vi "Main - Handle Flat BOM Drag&Drop.vi"(8 "error in (no error)":errorcluster, 10 "Drag&Drop Data":T2, 11 "TreeControl in":refnum<vi>) -> (0 "error out":errorcluster, 2 "Data":T1, 3 "Refresh Table":bool)   [LabVIEW 2018]
uses:
  TypeDef/Main - Handle Heirarchy Drag&Drop - Data.ctl
  TypeDef/Main - Handle Heirarchy Drag&Drop - States.ctl
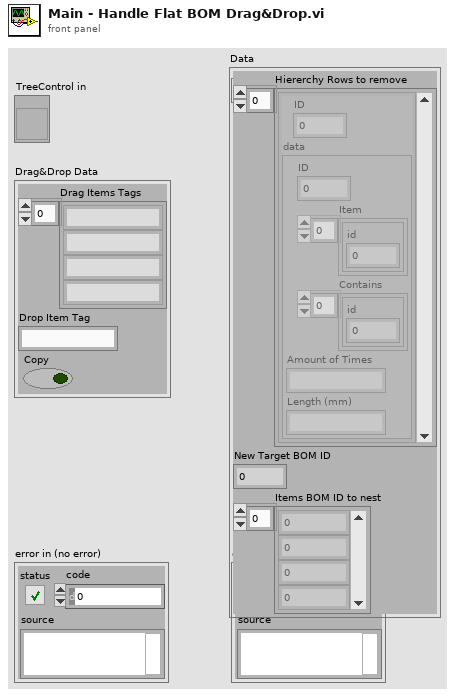
[diagram p1: front panel]
types:
  T1 = typedef "Main - Handle Heirarchy Drag&Drop - Data.ctl" = cluster{"Hiererchy Rows to remove":cluster{"ID":i32, "data":cluster{"ID":i32, "Item":cluster{"id":i32}[], "Contains":cluster{"id":i32}[], "Amount of Times":string, "Length (mm)":string}}[], "New Target BOM ID":i32, "Items BOM ID to nest":i32[]}
  T2 = cluster{"Drag Items Tags":string[], "Drop Item Tag":string, "Copy":bool}
  T3 = typedef "Main - Handle Heirarchy Drag&Drop - States.ctl" = enum16{"Check Data", "GET previous container entries", "Remove container entries", "Create new container entries", "Restore container entries", "Report Error", "Exit"}
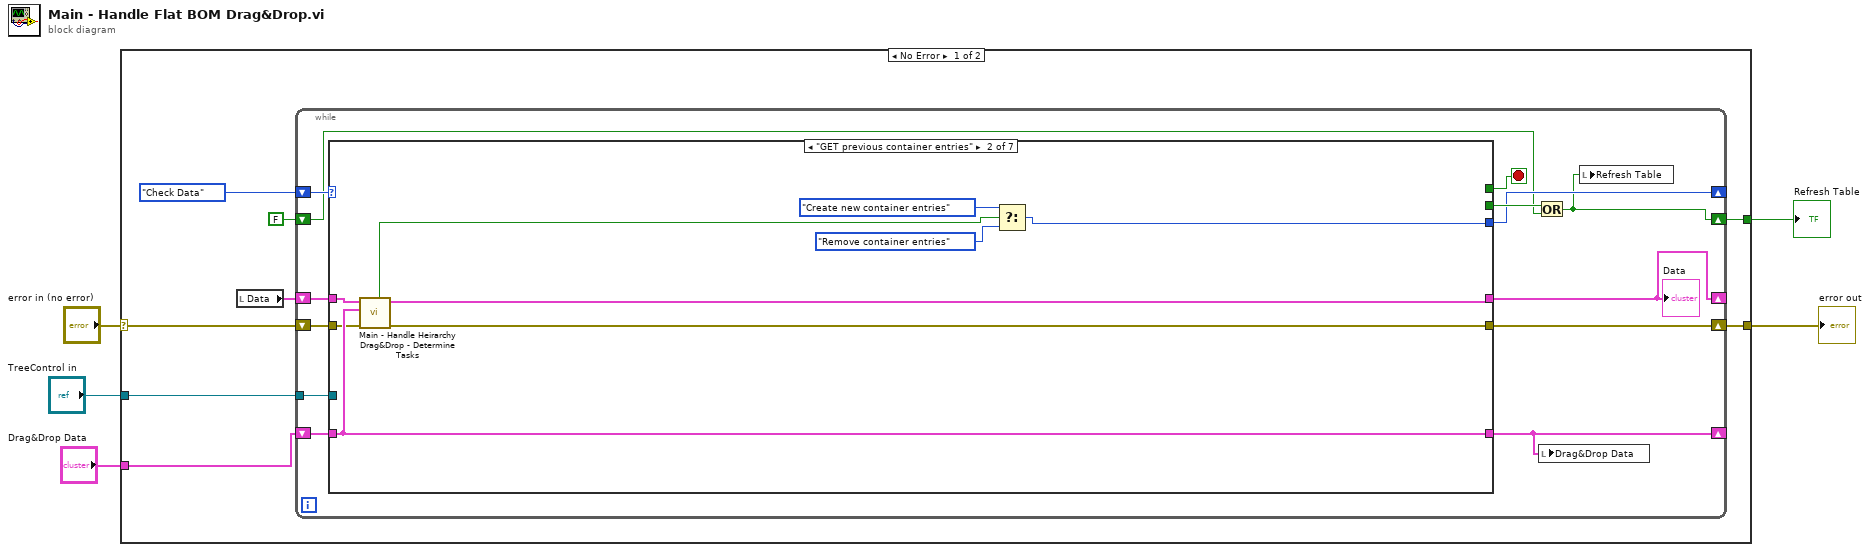
[diagram p0: block diagram]
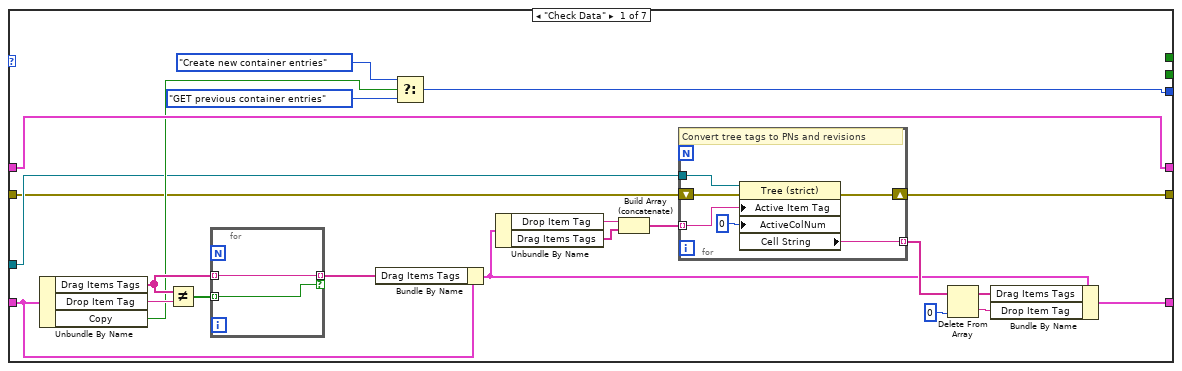
[diagram p2: hidden frame]
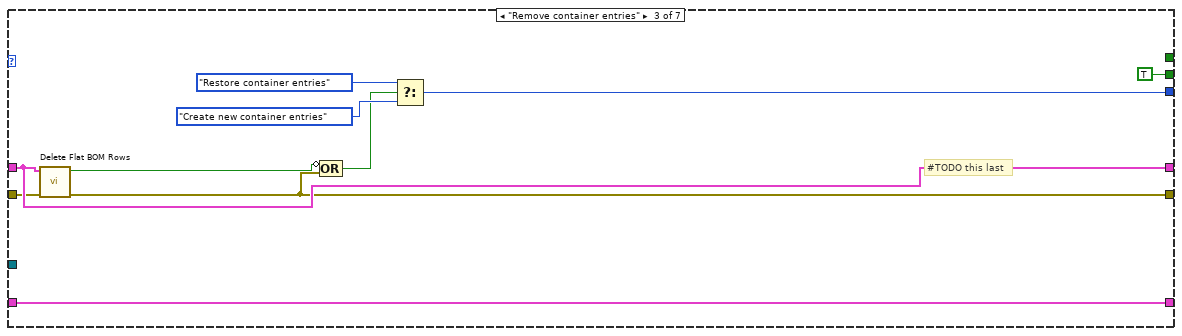
[diagram p3: hidden frame]
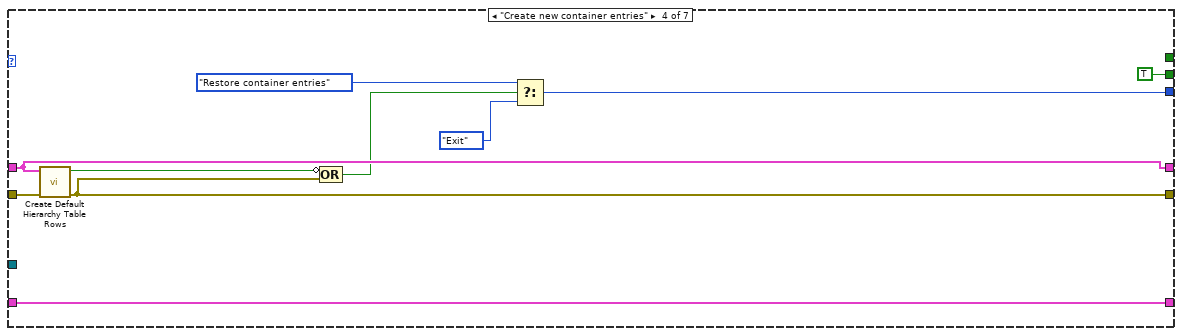
[diagram p4: hidden frame]
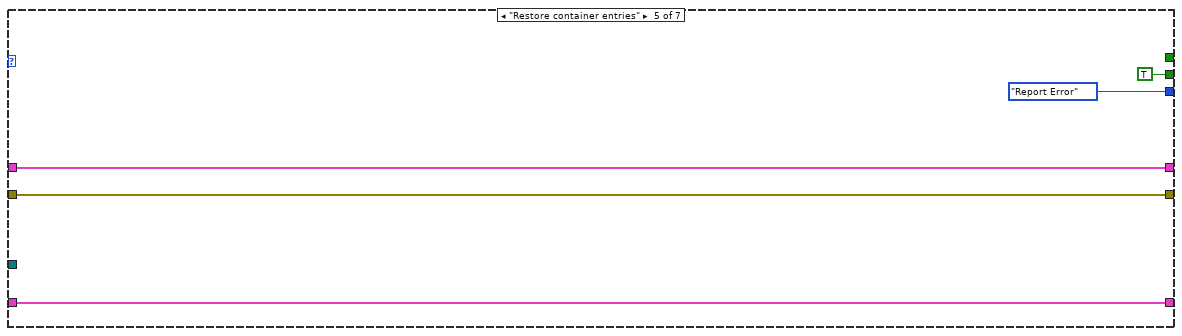
[diagram p5: hidden frame]
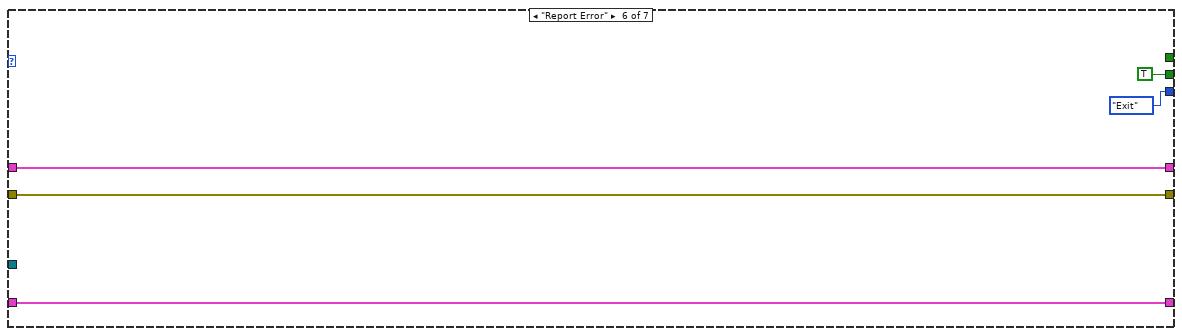
[diagram p6: hidden frame]
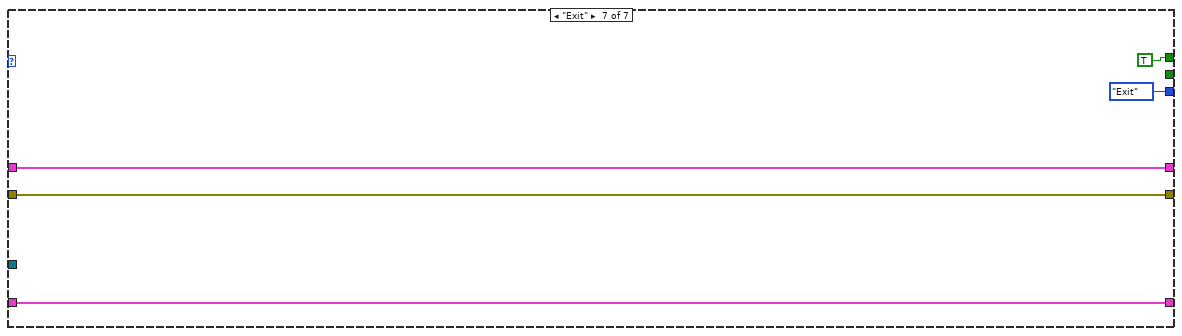
[diagram p7: hidden frame]
diagram:
  n1 = case shown="No Error" "error in (no error)" {
    selector: "error in (no error)" -> [w12 w101]
    tunnel: [w13 w101] -> w5
    tunnel: [w11 _] -> w3
    tunnel: "TreeControl in" -> [w10 _]
    tunnel: "Drag&Drop Data" -> [w9 _]
    frame No Error {
      n2 = local read "Data"() -> (w6:T1)
      n3 = while {
        tunnel: w10 -> [w23]
        shift-right: [w17] -> w11
        shift-left: FALSE -> [w18]
        shift-right: [w25] -> w13
        shift-left: w12 -> [w26]
        shift-right: [w19] -> _
        shift-left: Main_-_Handle_Heirarchy_Drag&Drop_-_States."Check Data" -> [w21]
        shift-right: [w16] -> _
        shift-left: w9 -> [w24]
        shift-right: [w15] -> _
        shift-left: w6 -> [w14]
        stop <- w20 stop-if-true
        n4 = case shown="\"GET previous container entries\"" w21 {
          tunnel: w26 -> [w28 w59 w68 w79 w90 w95 w99]
          tunnel: [w29 w60 w67 w76 w90 w95 w99] -> w25
          tunnel: w24 -> [w45 w63 w75 w85 w89 w94 w98]
          tunnel: w23 -> [w35 _ _ _ _ _ _]
          tunnel: [_ _ TRUE TRUE TRUE TRUE _] -> w22
          tunnel: [_ _ _ _ _ _ TRUE] -> w20
          tunnel: [w32 w63 w75 w85 w89 w94 w98] -> w16
          tunnel: [w40 w62 w72 w82 Main_-_Handle_Heirarchy_Drag&Drop_-_States."Report Error" Main_-_Handle_Heirarchy_Drag&Drop_-_States."Exit" Main_-_Handle_Heirarchy_Drag&Drop_-_States."Exit"] -> w19
          tunnel: w14 -> [w43 w61 w69 w80 w86 w91 w96]
          tunnel: [w43 w57 w69 w80 w86 w91 w96] -> w15
          frame "Check Data" {
            n5 = Unbundle By Name(w45) -> ("Drag Items Tags"=w47:string[], "Drop Item Tag"=w48:string, "Copy"=w42:bool)
            n6 = Not Equal?(x=w47, y=w48) -> (x != y?=w46:bool[])
            n7 = for {
              tunnel: w47 -> [w56] mode=indexing
              tunnel: [w56] -> w44 mode=indexing if=w55
              tunnel: w46 -> [w55] mode=indexing
            }
            n8 = Bundle By Name(cluster=w45, "Drag Items Tags"=w44) -> (w33:T2)
            n9 = Select(t=Main_-_Handle_Heirarchy_Drag&Drop_-_States."Create new container entries", s=w42, f=Main_-_Handle_Heirarchy_Drag&Drop_-_States."GET previous container entries") -> (s? t:f=w40:T3)
            n10 = Unbundle By Name(w33) -> ("Drop Item Tag"=w27:string, "Drag Items Tags"=w34:string[])
            n11 = Build Array (concatenate)(w27, w34) -> (w38:string[])
            n12 = for {
              tunnel: w35 -> [w54]
              tunnel: w38 -> [w53] mode=indexing
              tunnel: [w50] -> w37 mode=indexing
              shift-right: [w51] -> w29
              shift-left: w28 -> [w52]
              # "Convert tree tags to PNs and revisions"
              n13 = property class="Tree (strict)"(reference=w54, error in=w52, "Active Item Tag"=w53, "ActiveColNum"=0 ("Active Cell:Active Column Number")) -> (error out=w51:errorcluster, "Cell String"=w50:string)  [unwired: 1 out]
            }
            n14 = Delete From Array(array=w37, index=0) -> (deleted portion=w31:string, array with subset deleted=w30:string[])  [unwired: 1 in]
            n15 = Bundle By Name(cluster=w33, "Drag Items Tags"=w30, "Drop Item Tag"=w31) -> (w32:T2)
          }
          frame "GET previous container entries" {
            n16 = call "Main - Handle Heirarchy Drag&Drop - Determine Tasks.vi"("error in (no error)"=w59, "Drag&Drop Data"=w63, "Data in"=w61) -> ("error out"=w60:errorcluster, "Data out"=w57:T1, "Copy"=w58:bool)  [unwired: 6 in]
            n17 = Select(t=Main_-_Handle_Heirarchy_Drag&Drop_-_States."Create new container entries", s=w58, f=Main_-_Handle_Heirarchy_Drag&Drop_-_States."Remove container entries") -> (s? t:f=w62:T3)
          }
          frame "Remove container entries" {
            # "#TODO this last"
            n18 = call "Delete Flat BOM Rows.vi"("error in (no error)"=w68, "Data"=w69) -> ("error out"=w67:errorcluster, "OK"=w66:bool)  [unwired: 8 in]
            n19 = Compound Arithmetic op=OR(invert w66, w67) -> (w70:bool)
            n20 = Select(t=Main_-_Handle_Heirarchy_Drag&Drop_-_States."Restore container entries", s=w70, f=Main_-_Handle_Heirarchy_Drag&Drop_-_States."Create new container entries") -> (s? t:f=w72:T3)
          }
          frame "Create new container entries" {
            n21 = call "Create Default Hierarchy Table Rows.vi"("Error in"=w79, "Data"=w80) -> ("Error out"=w76:errorcluster, "OK"=w77:bool)  [unwired: 8 in]
            n22 = Compound Arithmetic op=OR(invert w77, w76) -> (w78:bool)
            n23 = Select(t=Main_-_Handle_Heirarchy_Drag&Drop_-_States."Restore container entries", s=w78, f=Main_-_Handle_Heirarchy_Drag&Drop_-_States."Exit") -> (s? t:f=w82:T3)
          }
          frame "Restore container entries" {
          }
          frame "Report Error" {
          }
          frame "Exit" {
          }
        }
        "Data" <- w15
        n24 = Or(x=w22, y=w18) -> (x .or. y?=w17:bool)
        n25 = local write "Drag&Drop Data"(w16) -> ()
        n26 = local write "Refresh Table"(w17) -> ()
      }
    }
    frame Error {
    }
  }
  "error out" <- w5
  "Refresh Table" <- w3
